vi "Accurate Measure With Setting_ver2.vi"(0 "DMM ref in":refnum<visa-resource-name>, 1 "Accurate Measure Setting":T1={"Enable DMM Relay"=FALSE, "Measure Current Only"=FALSE, [], "channel_count"=11}, 2 "P_current_count":i32, 3 "N_current_count":i32, 5 "DMM error in":errorcluster, 7 "Current Sense \nResitance Array":dbl[](array[numeric])=[1.0032214, 1.00250644, 1.00234822, 1.0040944, 1.0017711, 1.00229431, 1.00344206, 1.00482066, 1.00381056, 1.00290978, 1.00333016, 1.00367587], 9 "ESP32 ref in":refnum<visa-resource-name>, 11 "ESP32 error in":errorcluster, 12 "current_mode":u8[](array[numeric])=[0, 0, 0, 0, 0, 0, 0, 0, 0, 0, 0]) -> (4 "DMM ref out":refnum<visa-resource-name>, 6 "DMM error out":errorcluster, 8 "Accurate Data":dbl[](array[numeric]), 10 "ESP32 ref out":refnum<visa-resource-name>, 13 "time_out_count":i32, 14 "Standard Deviation of Data":dbl[](array[numeric]), 15 "ESP32 error out":errorcluster)   [LabVIEW 2023]
uses:
  <instrlib>/Agilent 3446X Series/Agilent 3446X Series.lvlib
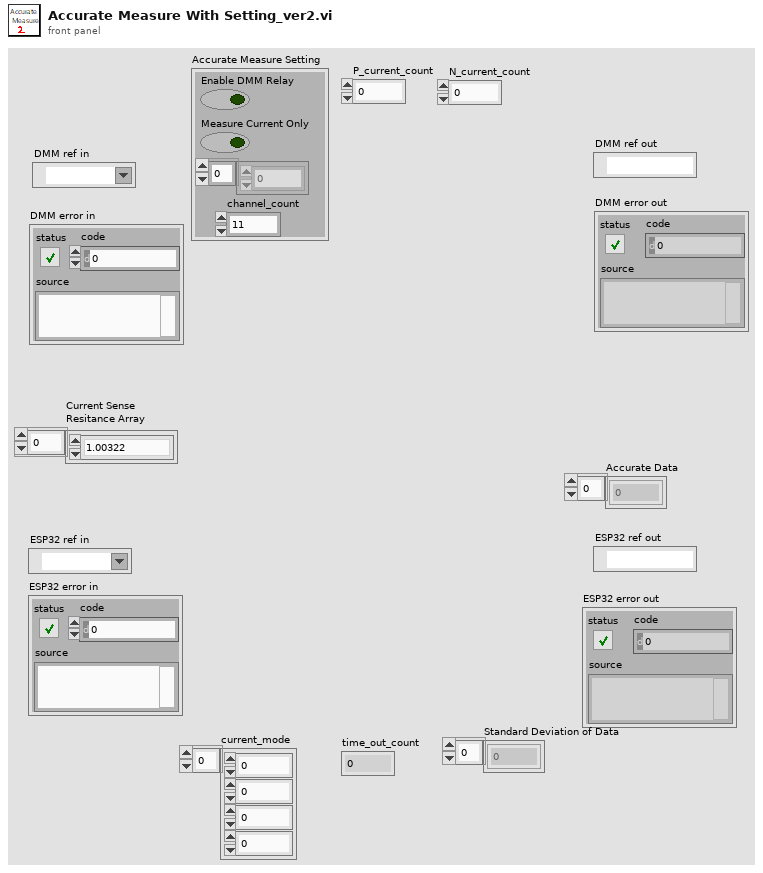
[diagram p1: front panel]
types:
  T1 = cluster{"Enable DMM Relay":bool, "Measure Current Only":bool, dbl[], "channel_count":i32}
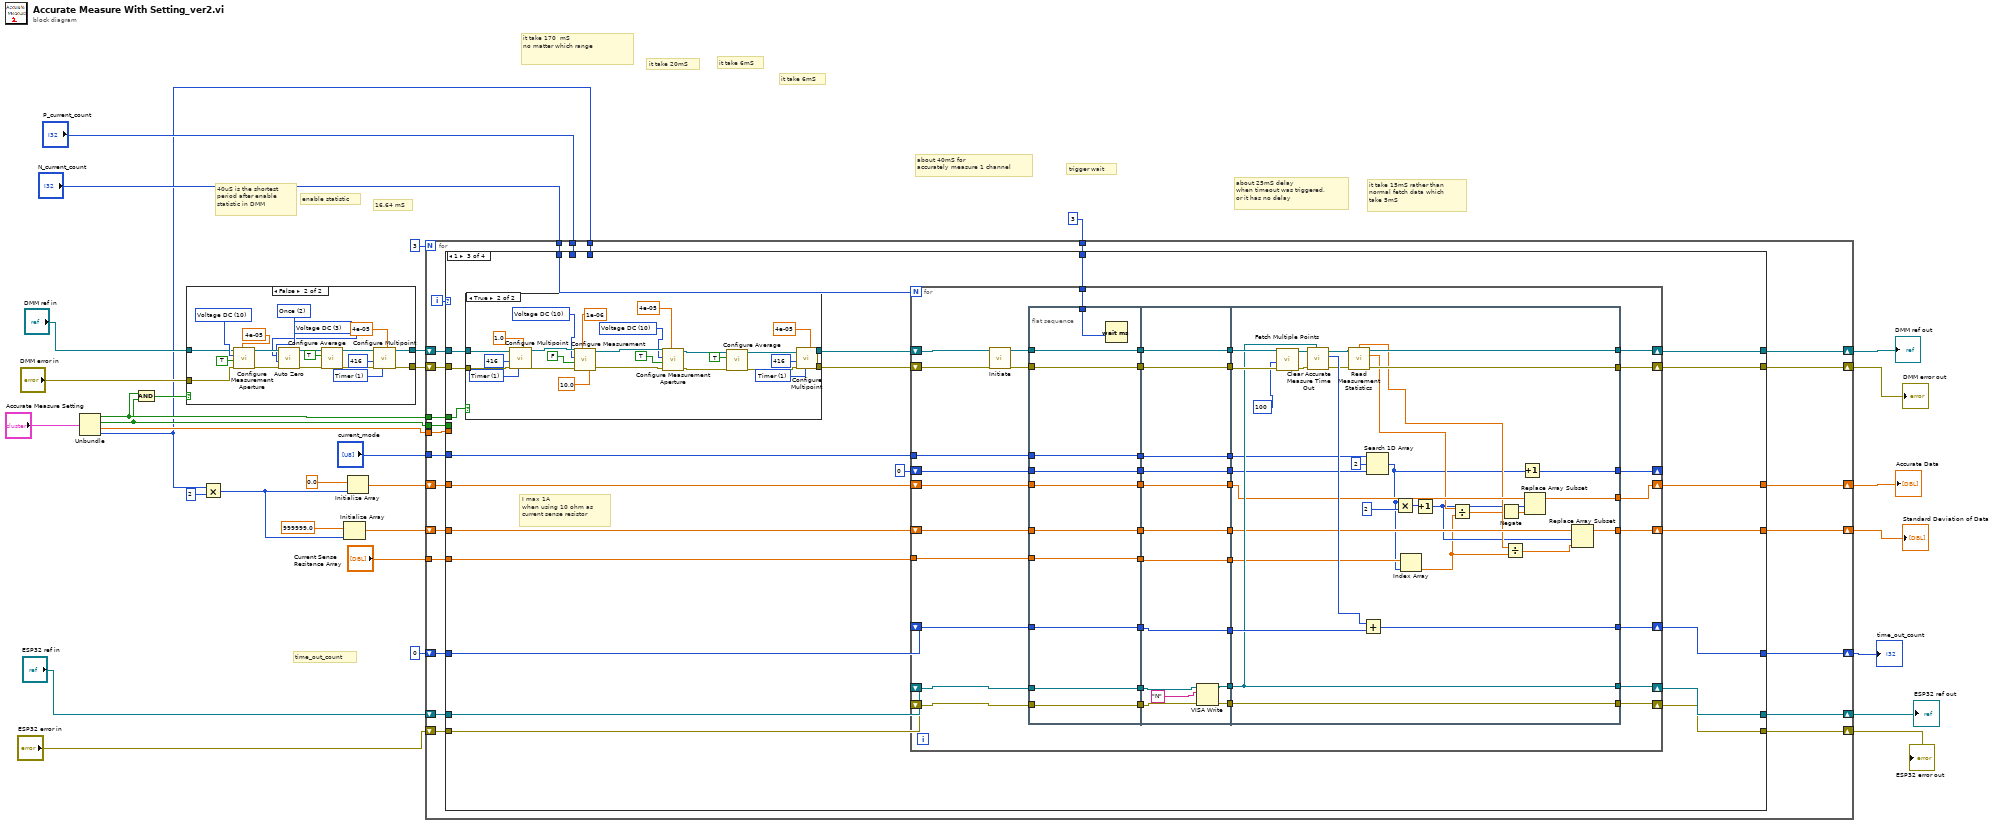
[diagram p0: block diagram]
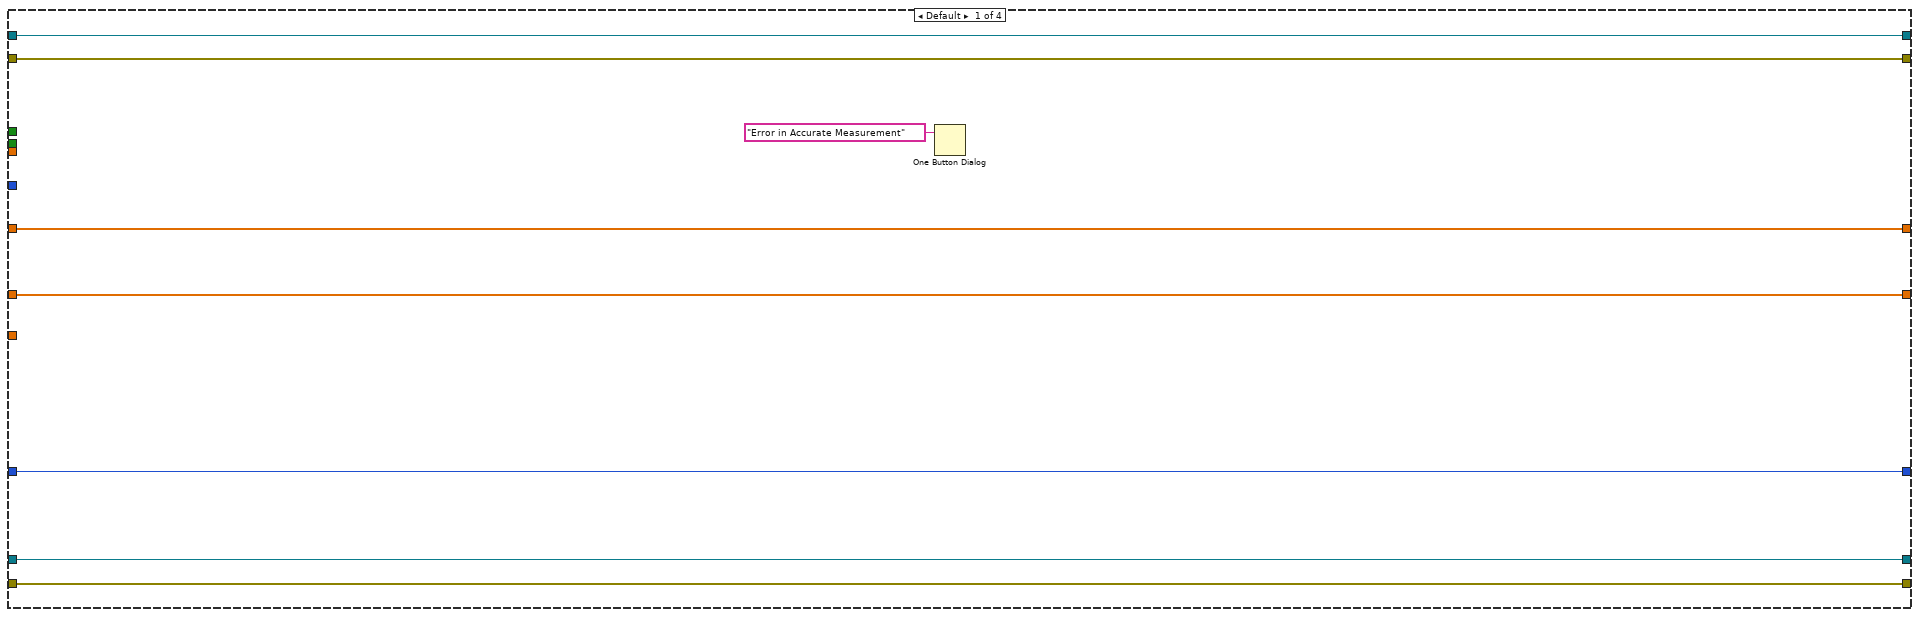
[diagram p3: hidden frame]
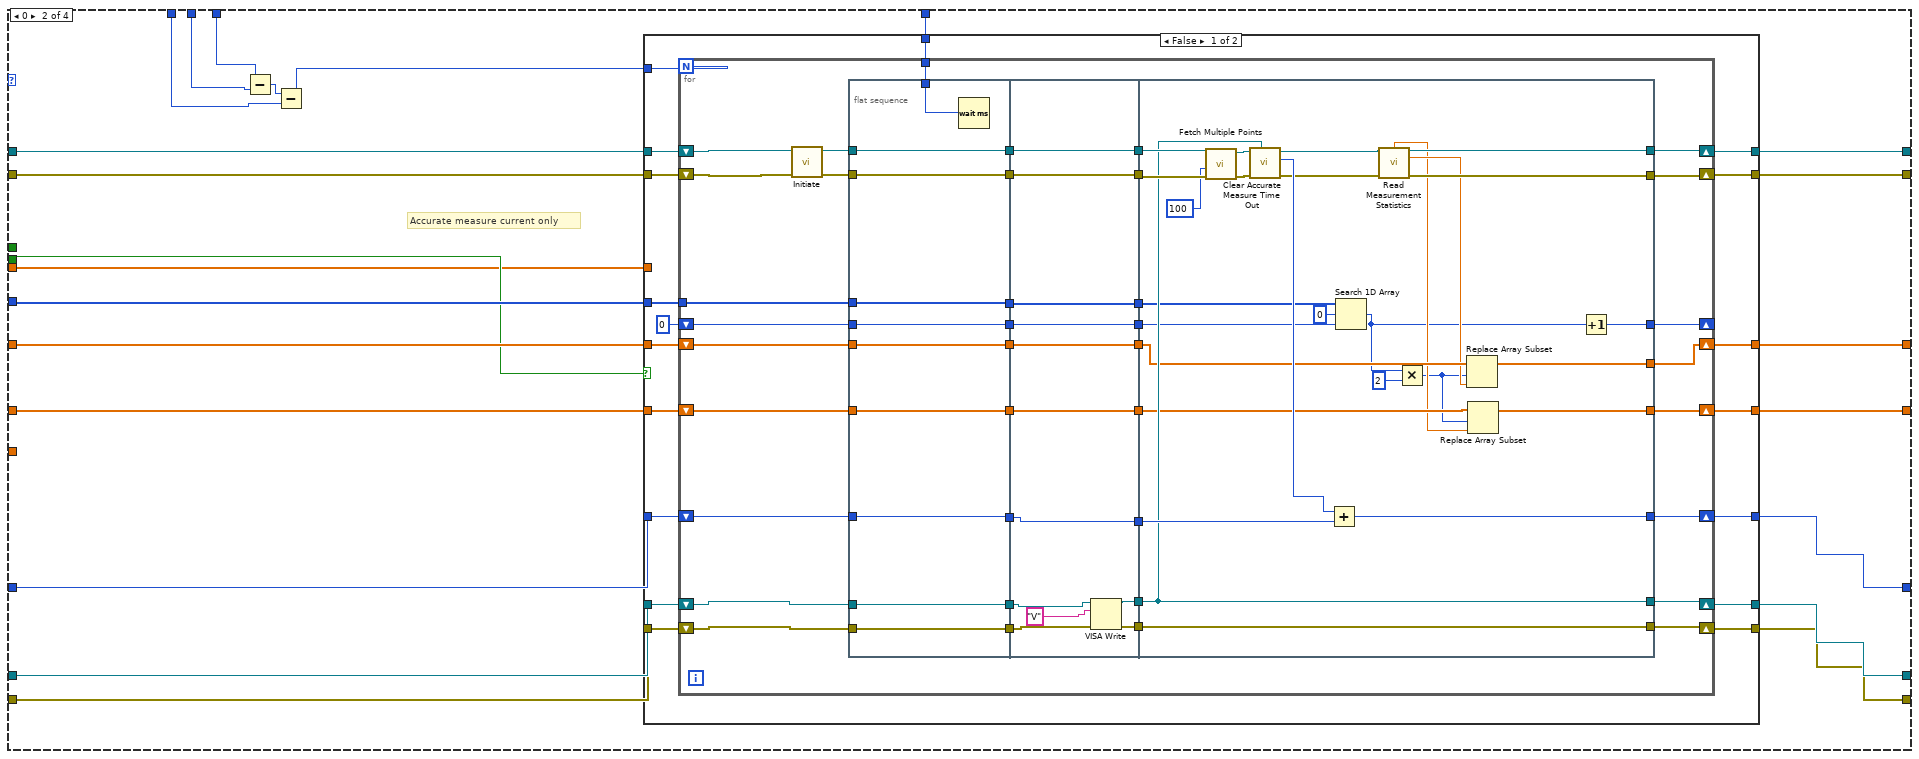
[diagram p4: hidden frame]
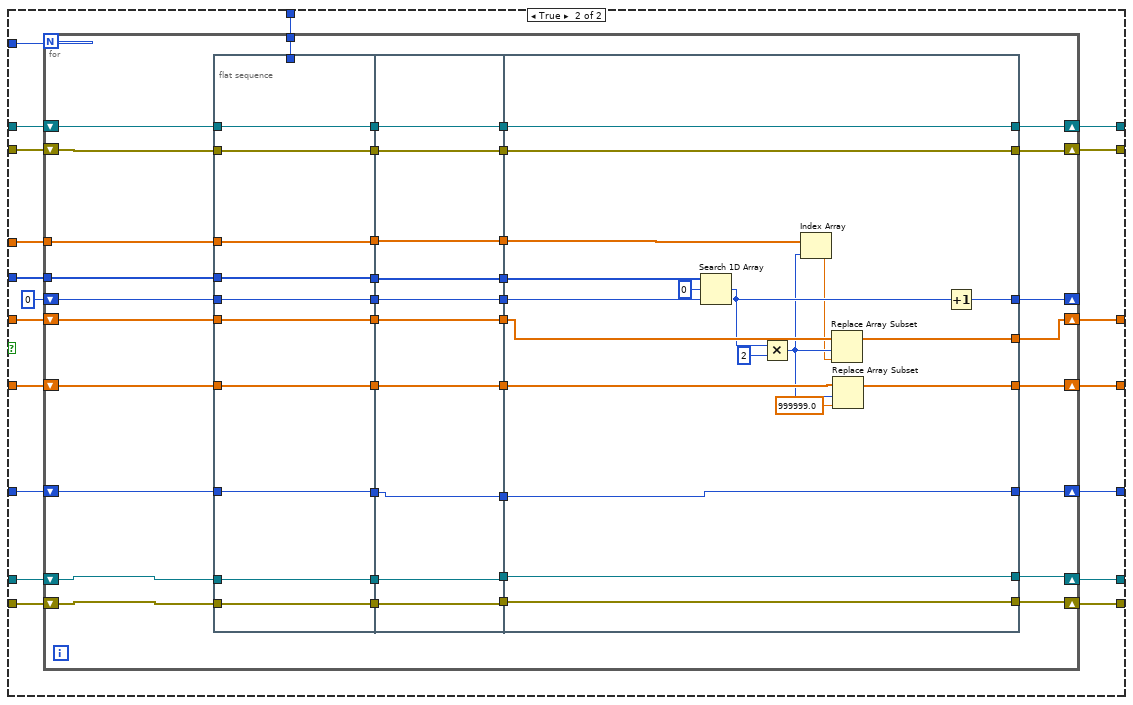
[diagram p5: hidden frame]
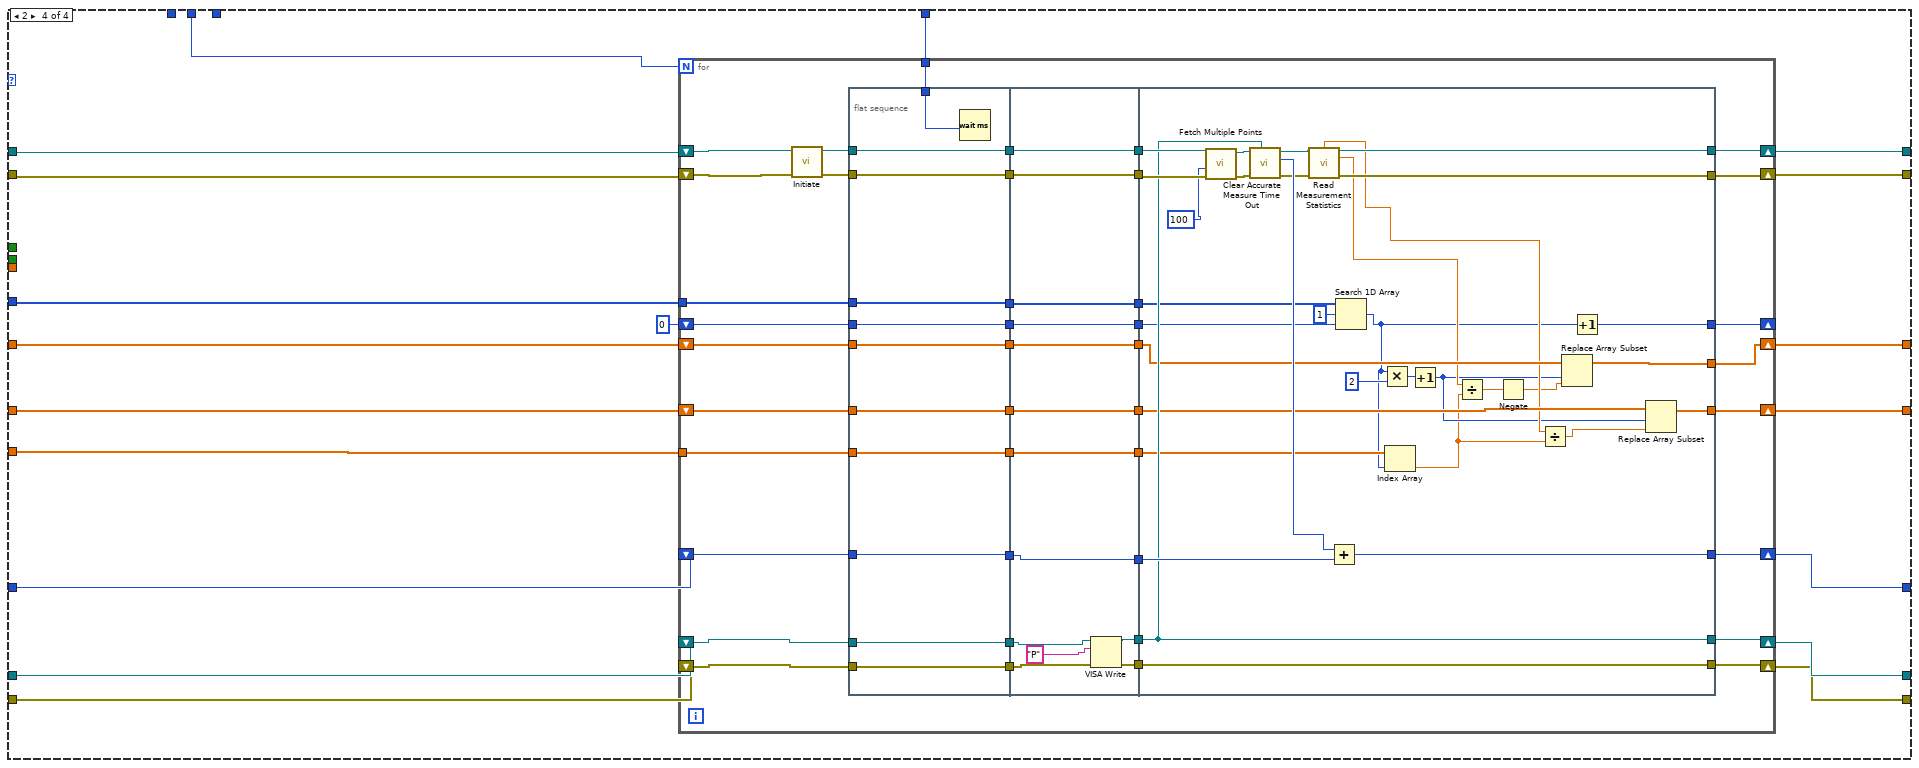
[diagram p7: hidden frame]
diagram:
  # "it take 6mS"
  # "it take 6mS"
  # "it take 20mS"
  # "it take 170  mS\nno matter which range"
  # "it take 15mS rather than\nnormal fetch data which \ntake 5mS"
  # "about 40mS for \naccurately measure 1 channel"
  # "about 25mS delay\nwhen timeout was triggered,\nor it has no delay"
  # "time_out_count"
  # "trigger wait"
  # "16.64 mS"
  # "enable statistic"
  # "40uS is the shortest\nperiod after enable \nstatistic in DMM"
  n1 = Unbundle("Accurate Measure Setting") -> ("Enable DMM Relay"=w5:bool, "Measure Current Only"=w4:bool, w6:dbl[], "channel_count"=w2:i32)
  n2 = And(x=w5, y=w4) -> (x .and. y?=w3:bool)
  n3 = case shown="False" w3 {
    tunnel: [w34 w38] -> w32
    tunnel: [w33 w37] -> w31
    tunnel: "DMM ref in" -> [w34 w36]
    tunnel: "DMM error in" -> [w33 w35]
    frame True {
    }
    frame False {
      w40 = 1 items=["Immediate", "Timer"] ("Sample Source (0: Immediate)")
      w47 = 3 items=["Current DC", "Resistance", "Temperature", "Voltage DC"] ("Zero Type (0: Current DC)")
      w48 = 2 items=["Disable", "Enable", "Once"] ("Auto Zero (1: Enable)")
      w44 = 10 items=["Continuity", "Current AC", "Current DC", "Diode", "Frequency", "Resistance 4-wire", "Period", "Resistance 2-wire", "Temperature", "Voltage AC", "Voltage DC", "Voltage DC Ratio", "Capacitance"] ("Measurement Function (0: Continuity)")
      n4 = call <instrlib>:"Configure Measurement Aperture.vi"("Aperture Time (0.1s)"=4e-05, "error in (no error)"=w35, "Enable Aperture (F: Disable)"=TRUE, "Measurement Function (0: Continuity)"=w44, "VISA resource name"=w36) -> ("error out"=w51:errorcluster, "VISA resource name out"=w50:refnum<visa-resource-name>)  [unwired: 5 in]
      n5 = call <instrlib>:"Auto Zero.vi"("error in (no error)"=w51, "Auto Zero (1: Enable)"=w48, "Zero Type (0: Current DC)"=w47, "VISA resource name"=w50) -> ("error out"=w53:errorcluster, "VISA resource name out"=w52:refnum<visa-resource-name>)  [unwired: 6 in]
      n6 = call <instrlib>:"Configure Average.vi"("error in (no error)"=w53, "Enable Statistics (F: Disable)"=TRUE, "VISA resource name"=w52) -> ("error out"=w42:errorcluster, "VISA resource name out"=w43:refnum<visa-resource-name>)  [unwired: 7 in]
      n7 = call <instrlib>:"Configure Multipoint.vi"("Sample Interval (1 Second)"=4e-05, "Sample Source (0: Immediate)"=w40, "error in (no error)"=w42, "Sample Count (1)"=416, "VISA resource name"=w43) -> ("error out"=w37:errorcluster, "VISA resource name out"=w38:refnum<visa-resource-name>)  [unwired: 2 in, 3 out]
    }
  }
  n8 = Multiply(x=w2, y=2) -> (x*y=w8:i32)
  n9 = Initialize Array(999999.0 ("Arithmetic Mean"), w8) -> (w17:dbl[])
  n10 = Initialize Array(0.0 ("Arithmetic Mean"), w8) -> (w20:dbl[])
  n11 = for {
    N: 3 -> [_]
    shift-right: [w75] -> w13
    shift-left: "ESP32 ref in" -> [w77]
    shift-right: [w74] -> w12
    shift-left: "ESP32 error in" -> [w76]
    shift-right: [w71] -> w15
    shift-left: w32 -> [w73]
    shift-right: [w70] -> w14
    shift-left: w31 -> [w72]
    tunnel: w2 -> [w69]
    tunnel: "P_current_count" -> [w68]
    tunnel: "N_current_count" -> [w67]
    tunnel: u32 3 ("milliseconds to wait") -> [w66]
    shift-right: [w65] -> w22
    shift-left: 0 -> [w64]
    shift-right: [w58] -> w11
    shift-left: w20 -> [w63]
    tunnel: "current_mode" -> [w62]
    shift-right: [w59] -> w10
    shift-left: w17 -> [w60]
    tunnel: w5 -> [w57]
    tunnel: w4 -> [w56]
    tunnel: w6 -> [w55]
    tunnel: "Current Sense \nResitance Array" -> [w54]
    i -> [w61]
    n12 = case shown="1" w61 {
      tunnel: w77 -> [w83 w104 w332 w477]
      tunnel: w76 -> [w82 w103 w331 w476]
      tunnel: [w83 w100 w328 w473] -> w75
      tunnel: [w82 w99 w327 w472] -> w74
      tunnel: w73 -> [w85 w106 w317 w462]
      tunnel: w72 -> [w84 w105 w316 w461]
      tunnel: [w85 w102 w330 w475] -> w71
      tunnel: [w84 w101 w329 w474] -> w70
      tunnel: w69 -> [_ w98 _ _]
      tunnel: w68 -> [_ w97 _ w459]
      tunnel: w67 -> [_ w96 w311 _]
      tunnel: [w79 w94 w325 w470] -> w65
      tunnel: w66 -> [_ w95 w326 w471]
      tunnel: w64 -> [w79 w93 w324 w469]
      tunnel: w63 -> [w81 w91 w322 w467]
      tunnel: w62 -> [_ w92 w323 w468]
      tunnel: w60 -> [w80 w90 w320 w465]
      tunnel: [w80 w89 w319 w464] -> w59
      tunnel: [w81 w88 w318 w463] -> w58
      tunnel: w57 -> [_ _ w313 _]
      tunnel: w56 -> [_ w87 _ _]
      tunnel: w55 -> [_ w86 _ _]
      tunnel: w54 -> [_ _ w312 w460]
      frame Default {
        n13 = One Button Dialog(message="Error in Accurate Measurement") -> ()  [unwired: 1 in, 1 out]
      }
      frame 0 {
        # "Accurate measure current only"
        n14 = Subtract(x=w98, y=w97) -> (x-y=w108:i32)
        n15 = Subtract(x=w108, y=w96) -> (x-y=w107:i32)
        n16 = case shown="False" w87 {
          tunnel: w107 -> [w126 w232]
          tunnel: w106 -> [w125 w231]
          tunnel: w105 -> [w124 w230]
          tunnel: w104 -> [w123 w229]
          tunnel: w103 -> [w122 w228]
          tunnel: [w121 w227] -> w102
          tunnel: [w120 w226] -> w101
          tunnel: [w119 w225] -> w100
          tunnel: [w118 w224] -> w99
          tunnel: w95 -> [w117 w223]
          tunnel: [w116 w222] -> w94
          tunnel: w93 -> [w115 w221]
          tunnel: w92 -> [w114 w220]
          tunnel: w91 -> [w113 w219]
          tunnel: w90 -> [w111 w217]
          tunnel: [w110 w216] -> w89
          tunnel: [w109 w215] -> w88
          tunnel: w86 -> [_ w214]
          frame False {
            n17 = for {
              N: w126 -> [_]
              shift-right: [w160] -> w121
              shift-left: w125 -> [w164]
              shift-right: [w159] -> w120
              shift-left: w124 -> [w163]
              shift-right: [w158] -> w119
              shift-left: w123 -> [w162]
              shift-right: [w157] -> w118
              shift-left: w122 -> [w161]
              tunnel: w117 -> [w143]
              shift-right: [w142] -> w116
              shift-left: w115 -> [w156]
              tunnel: w114 -> [w140]
              shift-right: [w128] -> w109
              shift-left: w113 -> [w137]
              shift-right: [w132] -> _
              shift-left: 0 ("index of element") -> [w133]
              shift-right: [w127] -> w110
              shift-left: w111 -> [w130]
              n18 = call <instrlib>:"Initiate.vi"("error in (no error)"=w163, "VISA resource name"=w164) -> ("error out"=w144:errorcluster, "VISA resource name out"=w145:refnum<visa-resource-name>)  [unwired: 8 in]
              n19 = flat-sequence {
                tunnel: [w174] -> w155
                tunnel: w162 -> [w174]
                tunnel: [w173] -> w154
                tunnel: w161 -> [w173]
                tunnel: w145 -> [w172]
                tunnel: [w172] -> w153
                tunnel: [w171] -> w152
                tunnel: w144 -> [w171]
                tunnel: [w170] -> w151
                tunnel: w156 -> [w170]
                tunnel: w143 -> [w169]
                tunnel: [w168] -> w141
                tunnel: w140 -> [w168]
                tunnel: [w167] -> w138
                tunnel: w137 -> [w167]
                tunnel: w133 -> [w166]
                tunnel: [w166] -> w135
                tunnel: [w165] -> w131
                tunnel: w130 -> [w165]
                tunnel: w155 -> [w186]
                tunnel: w154 -> [w185]
                tunnel: w153 -> [w184]
                tunnel: [w184] -> w147
                tunnel: w152 -> [w183]
                tunnel: [w183] -> w148
                tunnel: [w182] -> w149
                tunnel: [w181] -> w150
                tunnel: w151 -> [w179]
                tunnel: [w179] -> w146
                tunnel: w141 -> [w178]
                tunnel: [w178] -> w139
                tunnel: w138 -> [w177]
                tunnel: [w177] -> w136
                tunnel: w135 -> [w176]
                tunnel: [w176] -> w134
                tunnel: w131 -> [w175]
                tunnel: [w175] -> w129
                tunnel: [w213] -> w157
                tunnel: [w201] -> w158
                tunnel: [w205] -> w159
                tunnel: [w206] -> w160
                tunnel: w150 -> [w213]
                tunnel: w149 -> [w201]
                tunnel: w148 -> [w212]
                tunnel: w147 -> [w211]
                tunnel: [w207] -> w142
                tunnel: w146 -> [w202]
                tunnel: w139 -> [w200]
                tunnel: w136 -> [w196]
                tunnel: w134 -> [w198]
                tunnel: [w197] -> w132
                tunnel: w129 -> [w194]
                tunnel: [w192] -> w128
                tunnel: [w191] -> w127
                frame #0 {
                  n20 = Wait (ms)(milliseconds to wait=w169) -> ()  [unwired: 1 out]
                }
                frame #1 {
                  n21 = VISA Write(VISA resource name=w186, write buffer="V" ("data in"), error in (no error)=w185) -> (VISA resource name out=w182:refnum<visa-resource-name>, error out=w181:errorcluster)  [unwired: 1 out]
                }
                frame #2 {
                  n22 = call <instrlib>:"Fetch Multiple Points.vi"("error in (no error)"=w212, "Timeout (10000 ms)"=100, "VISA resource name"=w211) -> ("error out"=w209:errorcluster, "VISA resource name out"=w210:refnum<visa-resource-name>)  [unwired: 1 in, 6 out]
                  n23 = call "Clear Accurate Measure Time Out.vi"("ESP32 ref"=w201, "error in (no error)"=w209, "DMM ref"=w210) -> ("error out"=w203:errorcluster, "Time out count"=w208:i32, "VISA Refnum out"=w204:refnum<visa-resource-name>)  [unwired: 5 in, 1 out]
                  n24 = Add(x=w208, y=w202) -> (x+y=w207:i32)
                  n25 = Search 1D Array(1D array=w200, element=u8 0, start index (0)=w198) -> (index of element=w189:i32)
                  n26 = call <instrlib>:"Read Measurement Statistics.vi"("VISA resource name"=w204, "error in (no error)"=w203) -> ("Standard Deviation"=w193:dbl, "VISA resource name out"=w206:refnum<visa-resource-name>, "Arithmetic Mean"=w195:dbl, "error out"=w205:errorcluster)  [unwired: 6 in, 4 out]
                  n27 = Multiply(x=w189, y=2) -> (x*y=w187:i32)
                  n28 = Replace Array Subset(array=w196, new element=w195, index=w187) -> (w192:dbl[])
                  n29 = Replace Array Subset(array=w194, new element=w193, index=w187) -> (w191:dbl[])
                  n30 = Increment(x=w189) -> (x+1=w197:i32)
                }
              }
            }
          }
          frame True {
            n31 = for {
              N: w232 -> [_]
              shift-right: [w241] -> w227
              shift-left: w231 -> [w243]
              shift-right: [w236] -> w226
              shift-left: w230 -> [w238]
              shift-right: [w269] -> w225
              shift-left: w229 -> [w271]
              shift-right: [w268] -> w224
              shift-left: w228 -> [w270]
              tunnel: w223 -> [w260]
              shift-right: [w259] -> w222
              shift-left: w221 -> [w267]
              tunnel: w220 -> [w257]
              shift-right: [w245] -> w215
              shift-left: w219 -> [w254]
              shift-right: [w249] -> _
              shift-left: 0 ("index of element") -> [w250]
              shift-right: [w244] -> w216
              shift-left: w217 -> [w247]
              tunnel: w214 -> [w233]
              n32 = flat-sequence {
                tunnel: [w281] -> w266
                tunnel: w271 -> [w281]
                tunnel: [w280] -> w265
                tunnel: w270 -> [w280]
                tunnel: [w279] -> w264
                tunnel: w267 -> [w279]
                tunnel: w260 -> [_]
                tunnel: [w278] -> w258
                tunnel: w257 -> [w278]
                tunnel: [w277] -> w255
                tunnel: w254 -> [w277]
                tunnel: w250 -> [w276]
                tunnel: [w276] -> w252
                tunnel: [w275] -> w248
                tunnel: w247 -> [w275]
                tunnel: w243 -> [w274]
                tunnel: [w274] -> w240
                tunnel: [w273] -> w239
                tunnel: w238 -> [w273]
                tunnel: [w272] -> w235
                tunnel: w233 -> [w272]
                tunnel: w266 -> [w284]
                tunnel: w265 -> [w283]
                tunnel: [w284] -> w262
                tunnel: [w283] -> w263
                tunnel: w264 -> [w291]
                tunnel: [w291] -> w261
                tunnel: w258 -> [w290]
                tunnel: [w290] -> w256
                tunnel: w255 -> [w289]
                tunnel: [w289] -> w253
                tunnel: w252 -> [w288]
                tunnel: [w288] -> w251
                tunnel: w248 -> [w287]
                tunnel: [w287] -> w246
                tunnel: [w286] -> w242
                tunnel: w240 -> [w286]
                tunnel: w239 -> [w285]
                tunnel: [w285] -> w237
                tunnel: w235 -> [w282]
                tunnel: [w282] -> w234
                tunnel: [w310] -> w268
                tunnel: [w309] -> w269
                tunnel: w263 -> [w310]
                tunnel: w262 -> [w309]
                tunnel: [w292] -> w259
                tunnel: w261 -> [w292]
                tunnel: w256 -> [w308]
                tunnel: w253 -> [w304]
                tunnel: w251 -> [w306]
                tunnel: [w305] -> w249
                tunnel: w246 -> [w303]
                tunnel: [w302] -> w245
                tunnel: [w301] -> w244
                tunnel: w242 -> [w298]
                tunnel: [w298] -> w241
                tunnel: [w297] -> w236
                tunnel: w237 -> [w297]
                tunnel: w234 -> [w295]
                frame #0 {
                }
                frame #1 {
                }
                frame #2 {
                  n33 = Search 1D Array(1D array=w308, element=u8 0, start index (0)=w306) -> (index of element=w300:i32)
                  n34 = Multiply(x=w300, y=2) -> (x*y=w294:i32)
                  n35 = Index Array(array=w295, index=w294) -> (element=w293:dbl)
                  n36 = Replace Array Subset(array=w304, new element=w293, index=w294) -> (w302:dbl[])
                  n37 = Replace Array Subset(array=w303, new element=999999.0 ("new element/subarray"), index=w294) -> (w301:dbl[])
                  n38 = Increment(x=w300) -> (x+1=w305:i32)
                }
              }
            }
          }
        }
      }
      frame 1 {
        # "I max 1A\nwhen using 10 ohm as \ncurrent sense resistor"
        n39 = case shown="True" w313 {
          tunnel: w317 -> [w334 w340]
          tunnel: w316 -> [w333 w339]
          tunnel: [w334 w338] -> w315
          tunnel: [w333 w337] -> w314
          frame False {
          }
          frame True {
            w350 = 1 items=["Immediate", "Timer"] ("Sample Source (0: Immediate)")
            w346 = 10 items=["Continuity", "Current AC", "Current DC", "Diode", "Frequency", "Resistance 4-wire", "Period", "Resistance 2-wire", "Temperature", "Voltage AC", "Voltage DC", "Voltage DC Ratio", "Capacitance"] ("Measurement Function (0: Continuity)")
            w344 = 1 items=["Immediate", "Timer"] ("Sample Source (0: Immediate)")
            w341 = 10 items=["Continuity", "Current AC", "Current DC", "Diode", "Frequency", "Resistance 4-wire", "Period", "Resistance 2-wire", "Temperature", "Voltage AC", "Voltage DC", "Voltage DC Ratio", "Capacitance"] ("Measurement Function (10: Voltage DC)")
            n40 = call <instrlib>:"Configure Multipoint.vi"("Sample Interval (1 Second)"=1.0, "Sample Source (0: Immediate)"=w344, "error in (no error)"=w339, "Sample Count (1)"=416, "VISA resource name"=w340) -> ("error out"=w357:errorcluster, "VISA resource name out"=w356:refnum<visa-resource-name>)  [unwired: 2 in, 3 out]
            n41 = call <instrlib>:"Configure Measurement.vi"("Manual Range (1)"=10.0, "Absolute Resolution (1E-6)"=1e-06 ("x"), "error in (no error)"=w357, "Auto Range (T: Enable)"=FALSE, "Measurement Function (10: Voltage DC)"=w341, "VISA resource name"=w356) -> ("error out"=w354:errorcluster, "VISA resource name out"=w355:refnum<visa-resource-name>)  [unwired: 4 out]
            n42 = call <instrlib>:"Configure Measurement Aperture.vi"("Aperture Time (0.1s)"=4e-05, "error in (no error)"=w354, "Enable Aperture (F: Disable)"=TRUE, "Measurement Function (0: Continuity)"=w346, "VISA resource name"=w355) -> ("error out"=w359:errorcluster, "VISA resource name out"=w360:refnum<visa-resource-name>)  [unwired: 5 in]
            n43 = call <instrlib>:"Configure Average.vi"("error in (no error)"=w359, "Enable Statistics (F: Disable)"=TRUE, "VISA resource name"=w360) -> ("error out"=w358:errorcluster, "VISA resource name out"=w353:refnum<visa-resource-name>)  [unwired: 7 in]
            n44 = call <instrlib>:"Configure Multipoint.vi"("Sample Interval (1 Second)"=4e-05, "Sample Source (0: Immediate)"=w350, "error in (no error)"=w358, "Sample Count (1)"=416, "VISA resource name"=w353) -> ("error out"=w337:errorcluster, "VISA resource name out"=w338:refnum<visa-resource-name>)  [unwired: 2 in, 3 out]
          }
        }
        n45 = for {
          N: w311 -> [_]
          shift-right: [w397] -> w330
          shift-left: w315 -> [w401]
          shift-right: [w396] -> w329
          shift-left: w314 -> [w400]
          shift-right: [w395] -> w328
          shift-left: w332 -> [w399]
          shift-right: [w394] -> w327
          shift-left: w331 -> [w398]
          tunnel: w326 -> [w380]
          shift-right: [w379] -> w325
          shift-left: w324 -> [w393]
          tunnel: w323 -> [w377]
          shift-right: [w365] -> w318
          shift-left: w322 -> [w374]
          shift-right: [w369] -> _
          shift-left: 0 ("index of element") -> [w370]
          shift-right: [w364] -> w319
          shift-left: w320 -> [w367]
          tunnel: w312 -> [w362]
          n46 = call <instrlib>:"Initiate.vi"("error in (no error)"=w400, "VISA resource name"=w401) -> ("error out"=w381:errorcluster, "VISA resource name out"=w382:refnum<visa-resource-name>)  [unwired: 8 in]
          n47 = flat-sequence {
            tunnel: [w412] -> w392
            tunnel: w399 -> [w412]
            tunnel: [w411] -> w391
            tunnel: w398 -> [w411]
            tunnel: w382 -> [w410]
            tunnel: [w410] -> w390
            tunnel: [w409] -> w389
            tunnel: w381 -> [w409]
            tunnel: [w408] -> w388
            tunnel: w393 -> [w408]
            tunnel: w380 -> [w407]
            tunnel: [w406] -> w378
            tunnel: w377 -> [w406]
            tunnel: [w405] -> w375
            tunnel: w374 -> [w405]
            tunnel: w370 -> [w404]
            tunnel: [w404] -> w372
            tunnel: [w403] -> w368
            tunnel: w367 -> [w403]
            tunnel: [w402] -> w363
            tunnel: w362 -> [w402]
            tunnel: w392 -> [w425]
            tunnel: w391 -> [w424]
            tunnel: w390 -> [w423]
            tunnel: [w423] -> w384
            tunnel: w389 -> [w422]
            tunnel: [w422] -> w385
            tunnel: [w421] -> w386
            tunnel: [w420] -> w387
            tunnel: w388 -> [w418]
            tunnel: [w418] -> w383
            tunnel: w378 -> [w417]
            tunnel: [w417] -> w376
            tunnel: w375 -> [w416]
            tunnel: [w416] -> w373
            tunnel: w372 -> [w415]
            tunnel: [w415] -> w371
            tunnel: w368 -> [w414]
            tunnel: [w414] -> w366
            tunnel: w363 -> [w413]
            tunnel: [w413] -> w361
            tunnel: [w458] -> w394
            tunnel: [w446] -> w395
            tunnel: [w450] -> w396
            tunnel: [w451] -> w397
            tunnel: w387 -> [w458]
            tunnel: w386 -> [w446]
            tunnel: w385 -> [w457]
            tunnel: w384 -> [w456]
            tunnel: [w452] -> w379
            tunnel: w383 -> [w447]
            tunnel: w376 -> [w445]
            tunnel: w373 -> [w442]
            tunnel: w371 -> [w444]
            tunnel: [w443] -> w369
            tunnel: w366 -> [w441]
            tunnel: [w440] -> w365
            tunnel: [w439] -> w364
            tunnel: w361 -> [w435]
            frame #0 {
              n48 = Wait (ms)(milliseconds to wait=w407) -> ()  [unwired: 1 out]
            }
            frame #1 {
              n49 = VISA Write(VISA resource name=w425, write buffer="N" ("data in"), error in (no error)=w424) -> (VISA resource name out=w421:refnum<visa-resource-name>, error out=w420:errorcluster)  [unwired: 1 out]
            }
            frame #2 {
              n50 = call <instrlib>:"Fetch Multiple Points.vi"("error in (no error)"=w457, "Timeout (10000 ms)"=100, "VISA resource name"=w456) -> ("error out"=w454:errorcluster, "VISA resource name out"=w455:refnum<visa-resource-name>)  [unwired: 1 in, 6 out]
              n51 = call "Clear Accurate Measure Time Out.vi"("ESP32 ref"=w446, "error in (no error)"=w454, "DMM ref"=w455) -> ("error out"=w448:errorcluster, "Time out count"=w453:i32, "VISA Refnum out"=w449:refnum<visa-resource-name>)  [unwired: 5 in, 1 out]
              n52 = call <instrlib>:"Read Measurement Statistics.vi"("VISA resource name"=w449, "error in (no error)"=w448) -> ("Standard Deviation"=w437:dbl, "VISA resource name out"=w451:refnum<visa-resource-name>, "Arithmetic Mean"=w438:dbl, "error out"=w450:errorcluster)  [unwired: 6 in, 4 out]
              n53 = Add(x=w453, y=w447) -> (x+y=w452:i32)
              n54 = Search 1D Array(1D array=w445, element=u8 2, start index (0)=w444) -> (index of element=w430:i32)
              n55 = Multiply(x=w430, y=2) -> (x*y=w432:i32)
              n56 = Index Array(array=w435, index=w430) -> (element=w428:dbl)
              n57 = Increment(x=w432) -> (x+1=w431:i32)
              n58 = Divide(x=w438, y=w428) -> (x/y=w429:dbl)
              n59 = Negate(x=w429) -> (-x=w426:dbl)
              n60 = Divide(x=w437, y=w428) -> (x/y=w427:dbl)
              n61 = Increment(x=w430) -> (x+1=w443:i32)
              n62 = Replace Array Subset(array=w442, new element=w426, index=w431) -> (w440:dbl[])
              n63 = Replace Array Subset(array=w441, new element=w427, index=w431) -> (w439:dbl[])
            }
          }
        }
      }
      frame 2 {
        n64 = for {
          N: w459 -> [_]
          shift-right: [w514] -> w475
          shift-left: w462 -> [w518]
          shift-right: [w513] -> w474
          shift-left: w461 -> [w517]
          shift-right: [w512] -> w473
          shift-left: w477 -> [w516]
          shift-right: [w511] -> w472
          shift-left: w476 -> [w515]
          tunnel: w471 -> [w497]
          shift-right: [w496] -> w470
          shift-left: w469 -> [w510]
          tunnel: w468 -> [w494]
          shift-right: [w482] -> w463
          shift-left: w467 -> [w491]
          shift-right: [w486] -> _
          shift-left: 0 ("index of element") -> [w487]
          shift-right: [w481] -> w464
          shift-left: w465 -> [w484]
          tunnel: w460 -> [w479]
          n65 = call <instrlib>:"Initiate.vi"("error in (no error)"=w517, "VISA resource name"=w518) -> ("error out"=w498:errorcluster, "VISA resource name out"=w499:refnum<visa-resource-name>)  [unwired: 8 in]
          n66 = flat-sequence {
            tunnel: [w529] -> w509
            tunnel: w516 -> [w529]
            tunnel: [w528] -> w508
            tunnel: w515 -> [w528]
            tunnel: w499 -> [w527]
            tunnel: [w527] -> w507
            tunnel: [w526] -> w506
            tunnel: w498 -> [w526]
            tunnel: [w525] -> w505
            tunnel: w510 -> [w525]
            tunnel: w497 -> [w524]
            tunnel: [w523] -> w495
            tunnel: w494 -> [w523]
            tunnel: [w522] -> w492
            tunnel: w491 -> [w522]
            tunnel: w487 -> [w521]
            tunnel: [w521] -> w489
            tunnel: [w520] -> w485
            tunnel: w484 -> [w520]
            tunnel: [w519] -> w480
            tunnel: w479 -> [w519]
            tunnel: w509 -> [w542]
            tunnel: w508 -> [w541]
            tunnel: w507 -> [w540]
            tunnel: [w540] -> w501
            tunnel: w506 -> [w539]
            tunnel: [w539] -> w502
            tunnel: [w538] -> w503
            tunnel: [w537] -> w504
            tunnel: w505 -> [w535]
            tunnel: [w535] -> w500
            tunnel: w495 -> [w534]
            tunnel: [w534] -> w493
            tunnel: w492 -> [w533]
            tunnel: [w533] -> w490
            tunnel: w489 -> [w532]
            tunnel: [w532] -> w488
            tunnel: w485 -> [w531]
            tunnel: [w531] -> w483
            tunnel: w480 -> [w530]
            tunnel: [w530] -> w478
            tunnel: [w575] -> w511
            tunnel: [w563] -> w512
            tunnel: [w567] -> w513
            tunnel: [w568] -> w514
            tunnel: w504 -> [w575]
            tunnel: w503 -> [w563]
            tunnel: w502 -> [w574]
            tunnel: w501 -> [w573]
            tunnel: [w569] -> w496
            tunnel: w500 -> [w564]
            tunnel: w493 -> [w562]
            tunnel: w490 -> [w559]
            tunnel: w488 -> [w561]
            tunnel: [w560] -> w486
            tunnel: w483 -> [w558]
            tunnel: [w557] -> w482
            tunnel: [w556] -> w481
            tunnel: w478 -> [w552]
            frame #0 {
              n67 = Wait (ms)(milliseconds to wait=w524) -> ()  [unwired: 1 out]
            }
            frame #1 {
              n68 = VISA Write(VISA resource name=w542, write buffer="P" ("data in"), error in (no error)=w541) -> (VISA resource name out=w538:refnum<visa-resource-name>, error out=w537:errorcluster)  [unwired: 1 out]
            }
            frame #2 {
              n69 = call <instrlib>:"Fetch Multiple Points.vi"("error in (no error)"=w574, "Timeout (10000 ms)"=100, "VISA resource name"=w573) -> ("error out"=w571:errorcluster, "VISA resource name out"=w572:refnum<visa-resource-name>)  [unwired: 1 in, 6 out]
              n70 = call "Clear Accurate Measure Time Out.vi"("ESP32 ref"=w563, "error in (no error)"=w571, "DMM ref"=w572) -> ("error out"=w565:errorcluster, "Time out count"=w570:i32, "VISA Refnum out"=w566:refnum<visa-resource-name>)  [unwired: 5 in, 1 out]
              n71 = call <instrlib>:"Read Measurement Statistics.vi"("VISA resource name"=w566, "error in (no error)"=w565) -> ("Standard Deviation"=w554:dbl, "VISA resource name out"=w568:refnum<visa-resource-name>, "Arithmetic Mean"=w555:dbl, "error out"=w567:errorcluster)  [unwired: 6 in, 4 out]
              n72 = Add(x=w570, y=w564) -> (x+y=w569:i32)
              n73 = Search 1D Array(1D array=w562, element=u8 1, start index (0)=w561) -> (index of element=w547:i32)
              n74 = Multiply(x=w547, y=2) -> (x*y=w549:i32)
              n75 = Index Array(array=w552, index=w547) -> (element=w545:dbl)
              n76 = Increment(x=w549) -> (x+1=w548:i32)
              n77 = Divide(x=w555, y=w545) -> (x/y=w546:dbl)
              n78 = Negate(x=w546) -> (-x=w543:dbl)
              n79 = Divide(x=w554, y=w545) -> (x/y=w544:dbl)
              n80 = Replace Array Subset(array=w559, new element=w543, index=w548) -> (w557:dbl[])
              n81 = Increment(x=w547) -> (x+1=w560:i32)
              n82 = Replace Array Subset(array=w558, new element=w544, index=w548) -> (w556:dbl[])
            }
          }
        }
      }
    }
  }
  "time_out_count" <- w22
  "DMM ref out" <- w15
  "DMM error out" <- w14
  "ESP32 ref out" <- w13
  "ESP32 error out" <- w12
  "Accurate Data" <- w11
  "Standard Deviation of Data" <- w10
